vi "SDM Check Physical Channel Port.vi"(0 "Physical Channel In":tag, 11 "error in (no error)":errorcluster) -> (4 "Physical Channel Out":tag, 15 "error out":errorcluster)   [LabVIEW 2021, in "DAQ_Static Digital State Measurement.lvlib"]
doc: "Checks for the presence of port in the physical channel input and throws the required error when identified."
uses:
  DAQ_Static Digital State Measurement.lvlib
  <vilib>/Utility/error.llb/Error Cluster From Error Code.vi
  <vilib>/ErrorRing/Error Ring.xnode
  <resource>/objmgr/daqmx.rc
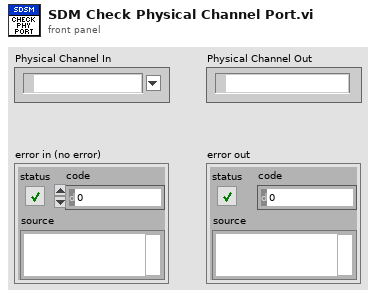
[diagram p1: front panel]
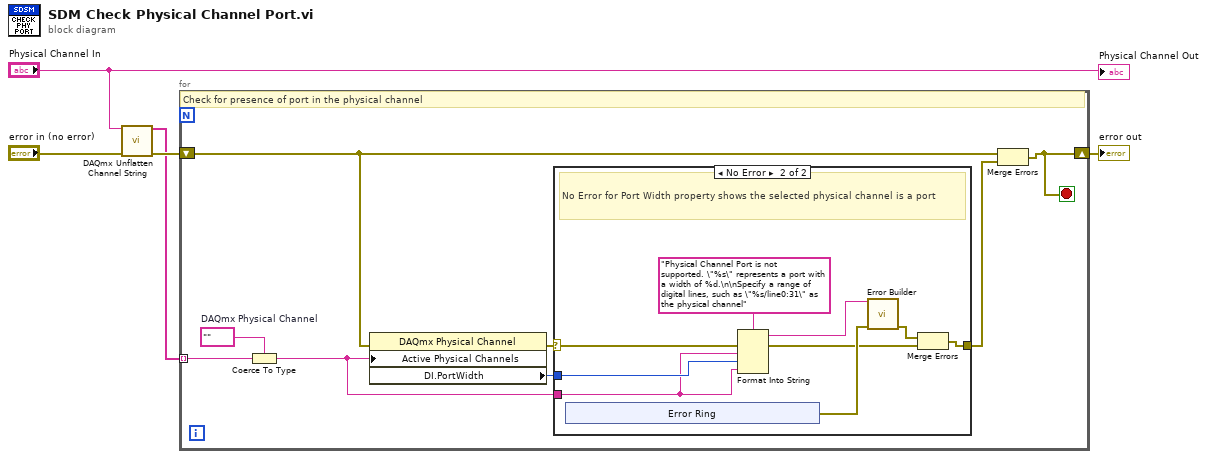
[diagram p0: block diagram]
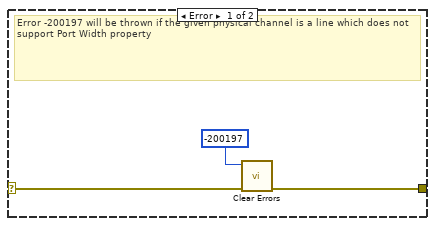
[diagram p2: hidden frame]
diagram:
  n1 = call <vilib>:"DAQmx Unflatten Channel String.vi"("names in"="Physical Channel In", "error in"="error in (no error)") -> ("names out"=w3:string[], "error out"=w4:errorcluster)  [unwired: 12 in]
  n2 = for {
    tunnel: w3 -> [w13] mode=indexing
    shift-right: [w9] -> w2
    shift-left: w4 -> [w11]
    stop <- w9 stop-if-true
    w12 = tag ""  # DAQmx Physical Channel
    # "Check for presence of port in the physical channel"
    n3 = Coerce To Type(0:w13, 1:w12) -> (2:w6:tag)
    n4 = property class="DAQmx Physical Channel"(error in=w11, "Active Physical Channels"=w6) -> (error out=w7:errorcluster, "DI.PortWidth"=w8:u32)  [unwired: 1 in, 1 out]
    n5 = case shown="No Error" w7 {
      selector: w7 -> [w16 w24]
      tunnel: [w15 w17] -> w10
      tunnel: w8 -> [_ w23]
      tunnel: w6 -> [_ w22]
      frame Error {
        # "Error -200197 will be thrown if the given physical channel is a line which does not support Port Width property"
        n6 = call <vilib>:"Clear Errors.vi"("error in (no error)"=w16, "specific error code to clear (0: all)"=-200197) -> ("error out"=w15:errorcluster)  [unwired: 4 in, 1 out]
      }
      frame No Error {
        # "No Error for Port Width property shows the selected physical channel is a port"
        n7 = xnode "Error Ring"() -> ("error out"=w20:errorcluster)
        n8 = Format Into String(format string="Physical Channel Port is not supported. \"%s\" represents a port with a width of %d.\n\nSpecify a range of digital lines, such as \"%s/line0:31\" as the physical channel" ("error message (\"\")"), error in=w24, w22, w23, w22) -> (resulting string=w21:string, error out=w18:errorcluster)  [unwired: 1 in]
        n9 = call "Error Builder.vi"("Error String"=w21, "Error In"=w20) -> ("Error Out"=w19:errorcluster)  [unwired: 13 in]
        n10 = Merge Errors(w19, w18) -> (w17:errorcluster)
      }
    }
    n11 = Merge Errors(w11, w10) -> (w9:errorcluster)
  }
  "error out" <- w2
  "Physical Channel Out" <- "Physical Channel In"
